vi "H5Tcreate.vi"(2 "size":i64, 7 "H5T_class_t":T1 items=["H5T_NO_CLASS"=-1, "H5T_INTEGER"=0, "H5T_FLOAT"=1, "H5T_TIME"=2, "H5T_STRING"=3, "H5T_BITFIELD"=4, "H5T_OPAQUE"=5, "H5T_COMPOUND"=6, "H5T_REFERENCE"=7, "H5T_ENUM"=8, "H5T_VLEN"=9, "H5T_ARRAY"=10], 9 "error in (no error)":errorcluster) -> (0 "datatype_id":i32, 6 "error out":errorcluster)   [LabVIEW 2009]
uses:
  H5T_class_t.ctl
  hdf5dll.dll
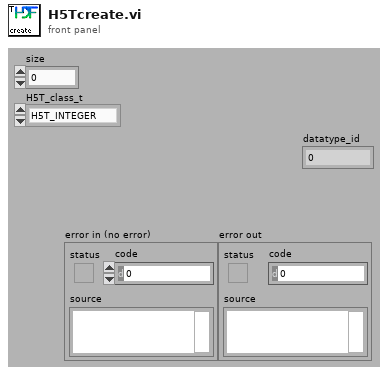
[diagram p1: front panel]
types:
  T1 = typedef "H5T_class_t.ctl" = i32
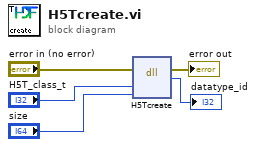
[diagram p0: block diagram]
diagram:
  n1 = dll-call lib="hdf5dll.dll" fn="H5Tcreate"(error in="error in (no error)", "class"="H5T_class_t", "size"="size") -> (error out=→"error out":errorcluster, "return type"=→"datatype_id":i32)  [unwired: 4 in, 1 out]
